vi "T to pH converter.vi"(1 "Waveform":dbl) -> (0 "Numeric":dbl)   [LabVIEW 2022 SP3]
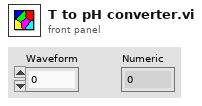
[diagram p1: front panel]
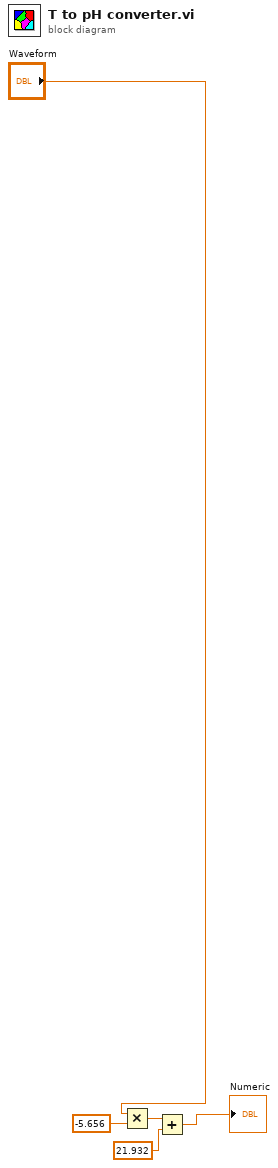
[diagram p0: block diagram]
diagram:
  n1 = Multiply(x="Waveform", y=-5.656) -> (x*y=w3:dbl)
  n2 = Add(x=w3, y=21.932) -> (x+y=→"Numeric":dbl)
